vi "GetParam.vi"(8 "error in (no error)":errorcluster caption="entrée d'erreur (pas d'erreur)", 11 "Kddcup99.lvclass":refnum<class "Kddcup99.lvclass">) -> (0 "error out":errorcluster caption="sortie d'erreur", 2 "fetch_kddcup99":T1={"subset"="None", "shuffle"=TRUE, "random_state"=-1, "percent10"=TRUE, "download_if_missing"=TRUE, "Returns"="Data"} {"random_state" min=-1}, 3 "Kddcup99.lvclass":refnum<class "Kddcup99.lvclass">)   [LabVIEW 2020, in "Kddcup99.lvclass"]
doc: "Get parameters"
uses:
  Kddcup99.lvclass
  Kddcup99.lvclass/Kddcup99.ctl
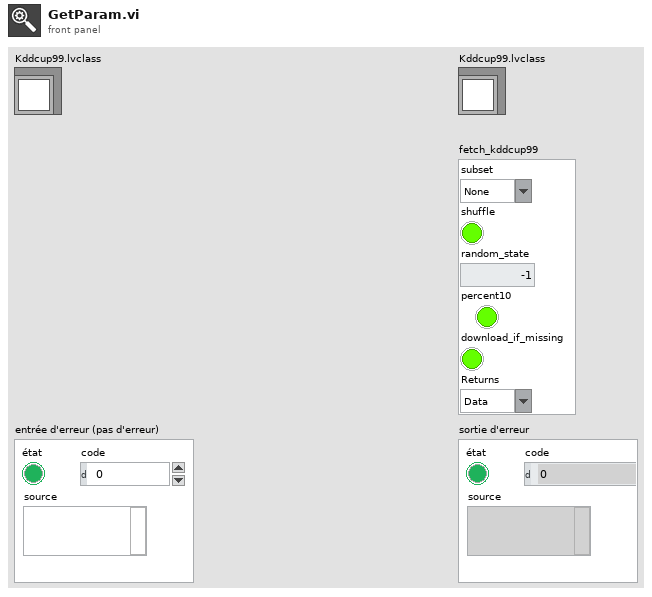
[diagram p1: front panel]
types:
  T1 = cluster{"subset":string, "shuffle":bool, "random_state":i32, "percent10":bool, "download_if_missing":bool, "Returns":string}
  T2 = cluster{"subset":string, "shuffle":bool, "random_state":i32, "percent10":bool, " download_if_missing ":bool, "Returns":string}
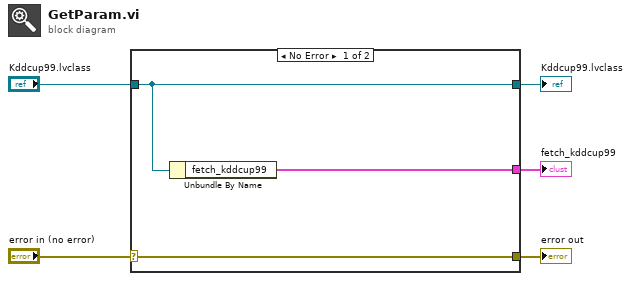
[diagram p0: block diagram]
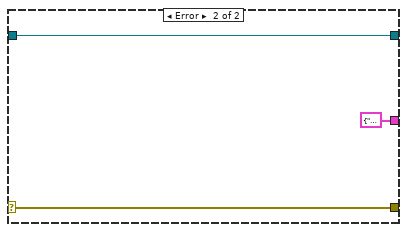
[diagram p2: hidden frame]
diagram:
  n1 = case shown="No Error" "error in (no error)" {
    selector: "error in (no error)" -> [w8 w10]
    tunnel: [w8 w10] -> w4
    tunnel: [w6 w11] -> w2
    tunnel: "Kddcup99.lvclass" -> [w6 w11]
    tunnel: [w7 T2 {"subset"="", "shuffle"=FALSE, "random_state"=0, "percent10"=FALSE, " download_if_missing "=FALSE, "Returns"=""} ("fetch_kddcup99")] -> w1
    frame No Error {
      n2 = Unbundle By Name(w6) -> ("fetch_kddcup99"=w7:T2)
    }
    frame Error {
    }
  }
  "error out" <- w4
  "Kddcup99.lvclass" <- w2
  "fetch_kddcup99" <- w1
